vi "Stare.vi"() -> ()   [LabVIEW 2020]
uses:
  <vilib>/ErrorRing/Error Ring.xnode
panel:
  in  "Combo Box":string(combo)
  out "Array 2":bool[](array[boolean])
  out "Array":dbl[](array[slide]) scale=0.0..100.0
  in  "alarma":dbl(slide) scale=0.0..100.0
  out "Estado":string
  in  "Data_Analisis.NombreArchivo":string
  in  "Data_Analisis.Direccion":path
  in  "Stop":bool
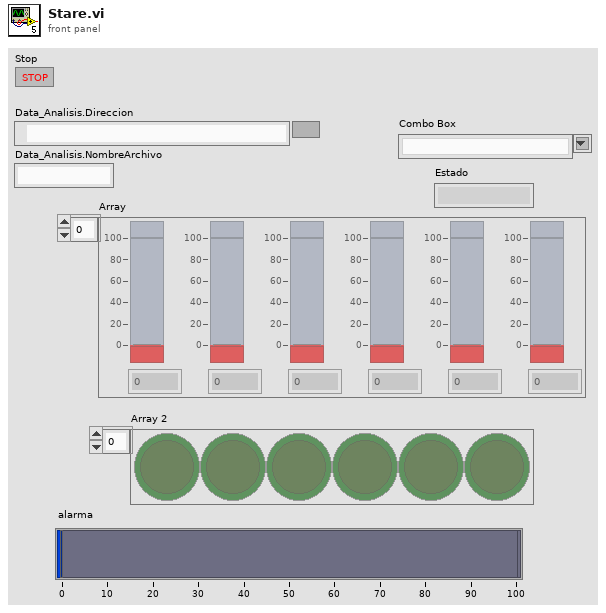
[diagram p1: front panel]
types:
  T1 = cluster{"Data_Analisis":cluster{"Direccion":path, "NombreArchivo":string, "Formato":string, "refnum out":refnum<file>}, "N_Values":cluster{"N_elementos":i32, "L_max":dbl, "L_min":dbl}, "Hardware":cluster{"Data_value":dbl[]}, "Alarmas":cluster{"Warning":bool[]}}
  T2 = cluster{"N_elementos":i32, "L_max":dbl, "L_min":dbl}
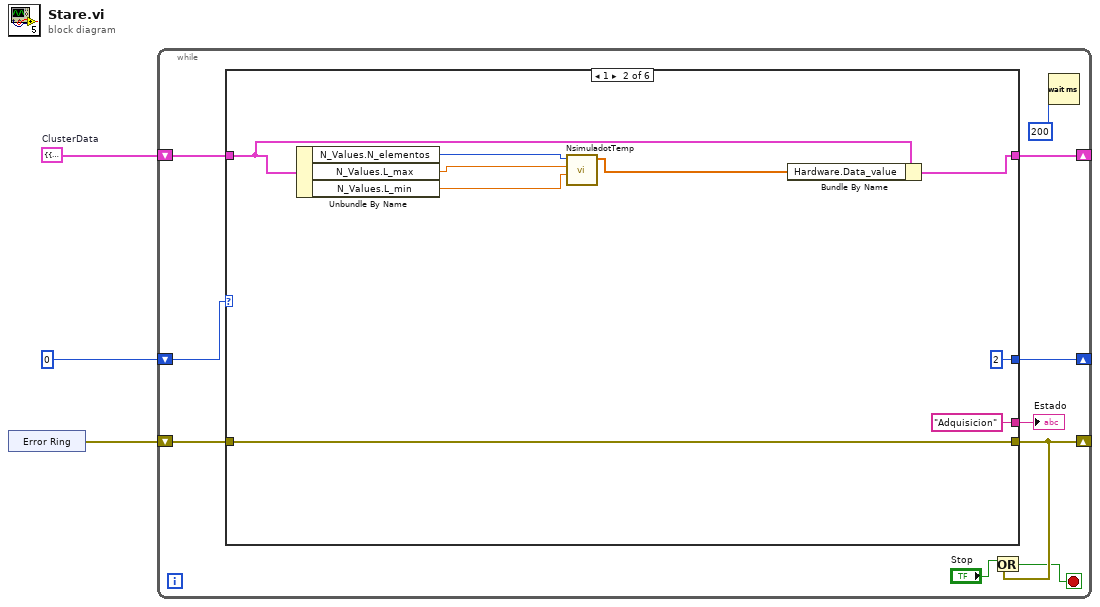
[diagram p0: block diagram]
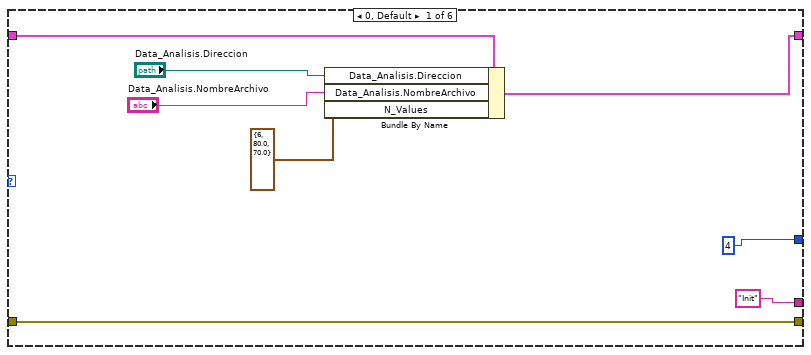
[diagram p2: hidden frame]
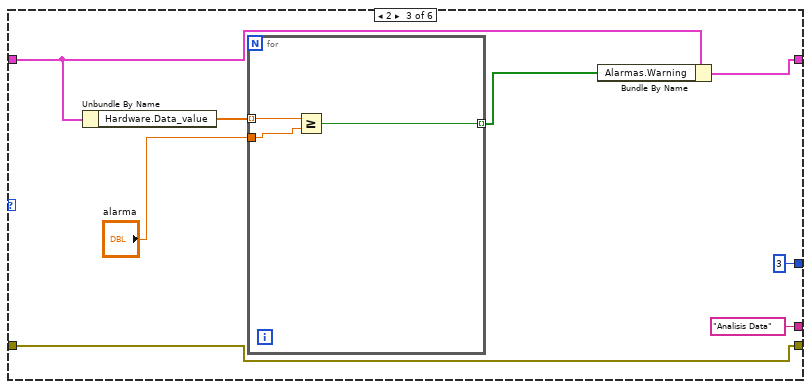
[diagram p3: hidden frame]
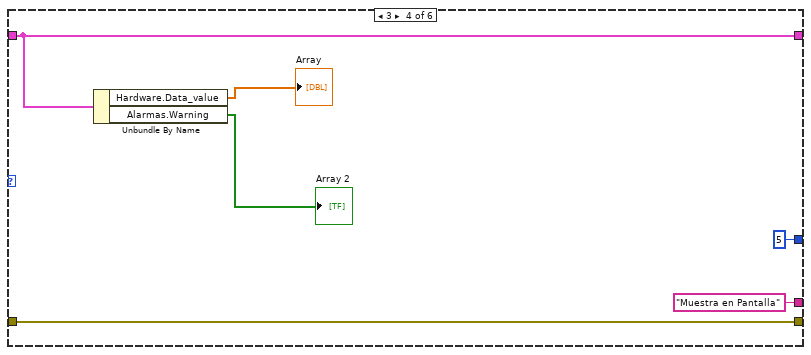
[diagram p4: hidden frame]
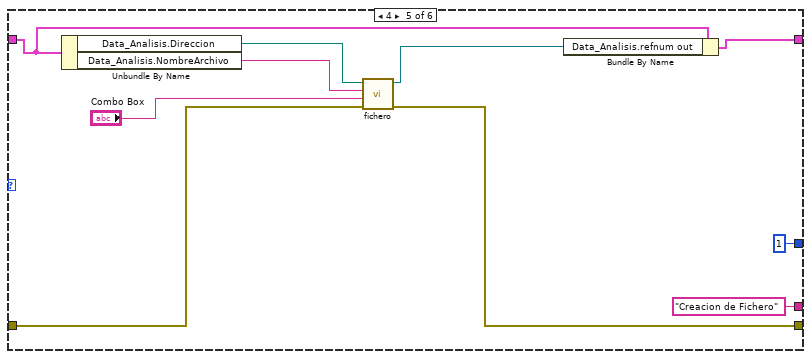
[diagram p5: hidden frame]
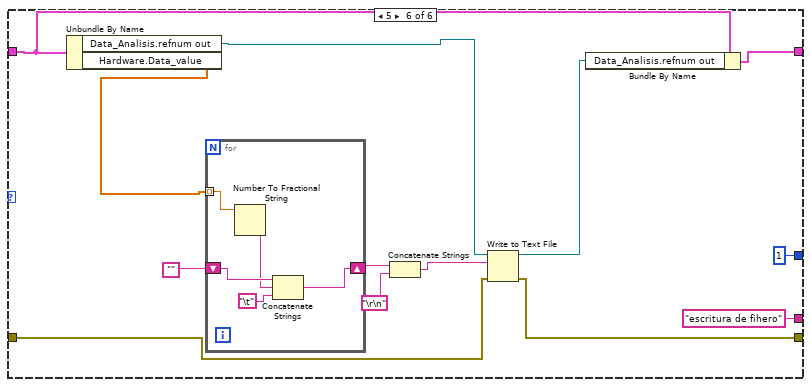
[diagram p6: hidden frame]
diagram:
  w3 = T1 {"Data_Analisis"={"Direccion"=path "", "NombreArchivo"="", "Formato"="", "refnum out"=refnum}, "N_Values"={"N_elementos"=0, "L_max"=0.0, "L_min"=0.0}, "Hardware"={"Data_value"=[]}, "Alarmas"={"Warning"=[FALSE]}}  # ClusterData
  n1 = xnode "Error Ring"() -> ("error out"=w1:errorcluster)
  n2 = while {
    shift-right: [w11] -> _
    shift-left: w3 -> [w12]
    shift-right: [w10] -> _
    shift-left: 0 -> [w13]
    shift-right: [w5] -> _
    shift-left: w1 -> [w8]
    stop <- w4 stop-if-true
    n3 = case shown="1" w13 {
      tunnel: w12 -> [w21 w27 w36 w47 w53 w62]
      tunnel: [w20 w25 w34 w47 w51 w60] -> w11
      tunnel: [4 2 3 5 1 1] -> w10
      tunnel: ["Init" ("Estado") "Adquisicion" ("Estado") "Analisis Data" ("Estado") "Muestra en Pantalla" ("Estado") "Creacion de Fichero" ("Estado") "escritura de fihero" ("Estado")] -> w9
      tunnel: [w14 w22 w32 w44 w54 w63] -> w5
      tunnel: w8 -> [w14 w22 w32 w44 w55 w64]
      frame 0, Default {
        n4 = Bundle By Name(cluster=w21, "Data_Analisis.Direccion"="Data_Analisis.Direccion", "Data_Analisis.NombreArchivo"="Data_Analisis.NombreArchivo", "N_Values"=T2 {"N_elementos"=6, "L_max"=80.0, "L_min"=70.0}) -> (w20:T1)
      }
      frame 1 {
        n5 = Unbundle By Name(w27) -> ("N_Values.N_elementos"=w30:i32, "N_Values.L_max"=w29:dbl, "N_Values.L_min"=w28:dbl)
        n6 = call "NsimuladotTemp.vi"("Lmin"=w28, "Lmax"=w29, "N"=w30) -> ("Array"=w26:dbl[])  [unwired: 8 in]
        n7 = Bundle By Name(cluster=w27, "Hardware.Data_value"=w26) -> (w25:T1)
      }
      frame 2 {
        n8 = Unbundle By Name(w36) -> ("Hardware.Data_value"=w38:dbl[])
        n9 = for {
          tunnel: w38 -> [w41] mode=indexing
          tunnel: "alarma" -> [w40]
          tunnel: [w39] -> w35 mode=indexing
          n10 = Greater Or Equal?(x=w41, y=w40) -> (x >= y?=w39:bool)
        }
        n11 = Bundle By Name(cluster=w36, "Alarmas.Warning"=w35) -> (w34:T1)
      }
      frame 3 {
        n12 = Unbundle By Name(w47) -> ("Hardware.Data_value"=→"Array":dbl[], "Alarmas.Warning"=→"Array 2":bool[])
      }
      frame 4 {
        n13 = Unbundle By Name(w53) -> ("Data_Analisis.Direccion"=w57:path, "Data_Analisis.NombreArchivo"=w56:string)
        n14 = call "fichero.vi"("error in (no error)"=w55, "Formato"="Combo Box", "Nombre"=w56, "Direccion"=w57) -> ("error out"=w54:errorcluster, "Byte Stream File out"=w52:refnum<file>)  [unwired: 6 in]
        n15 = Bundle By Name(cluster=w53, "Data_Analisis.refnum out"=w52) -> (w51:T1)
      }
      frame 5 {
        n16 = Unbundle By Name(w62) -> ("Data_Analisis.refnum out"=w66:refnum<file>, "Hardware.Data_value"=w70:dbl[])
        n17 = for {
          tunnel: w70 -> [w75] mode=indexing
          shift-right: [w71] -> w68
          shift-left: "" -> [w74]
          n18 = Number To Fractional String(number=w75) -> (F-format string=w73:string)  [unwired: 3 in]
          n19 = Concatenate Strings(w74, w73, "\t") -> (w71:string)
        }
        n20 = Concatenate Strings(w68, "\r\n") -> (w65:string)
        n21 = Write to Text File(file (use dialog)=w66, text=w65, error in=w64) -> (refnum out=w61:refnum<file>, error out=w63:errorcluster)  [unwired: 1 in, 1 out]
        n22 = Bundle By Name(cluster=w62, "Data_Analisis.refnum out"=w61) -> (w60:T1)
      }
    }
    "Estado" <- w9
    n23 = Or(x="Stop", y=w5) -> (x .or. y?=w4:bool)
    n24 = Wait (ms)(milliseconds to wait=u32 200) -> ()  [unwired: 1 out]
  }
